vi "WriteSystemData.vi"(8 "error in (no error)":errorcluster, 10 "SystemData":T1 {"SourceSelect" items=["儀器1"]}, 11 "DataNotifierIn":refnum<notifier>) -> (0 "error out":errorcluster, 3 "DataNotifierOut":refnum<notifier>)   [LabVIEW 2013, in "SystemData.lvclass"]
uses:
  SystemData.lvclass
  SystemDataTypeDefine.ctl
  Generator.lvclass/Generator.lvclass
  SystemData.lvclass/SystemData.ctl
panel:
  # "以notifier包裝systemData物件的參考\n如此不論在何處只要輸入正確notifier 參考\n就可以正確提出systemData物件保存的資料"
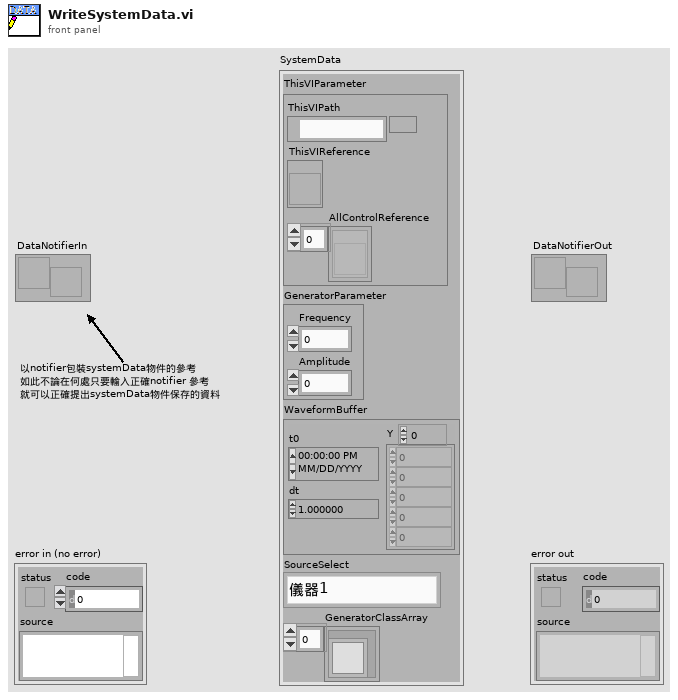
[diagram p1: front panel]
types:
  T1 = typedef "SystemData.lvclass/SystemDataTypeDefine.ctl" = cluster{"ThisVIParameter":cluster{"ThisVIPath":path, "ThisVIReference":refnum<vi>, "AllControlReference":refnum<vi>[]}, "GeneratorParameter":cluster{"Frequency":dbl, "Amplitude":dbl}, "WaveformBuffer":waveform(dbl), "SourceSelect":u16, "GeneratorClassArray":refnum<class "Generator.lvclass">[]}
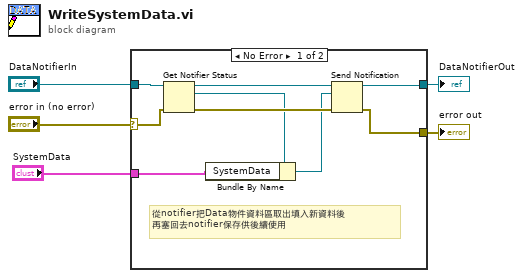
[diagram p0: block diagram]
diagram:
  n1 = case shown="No Error" "error in (no error)" {
    selector: "error in (no error)" -> [w10 w15]
    tunnel: [w9 w15] -> w4
    tunnel: [w11 w16] -> w2
    tunnel: "DataNotifierIn" -> [w14 w16]
    tunnel: "SystemData" -> [w7 _]
    frame No Error {
      # "從notifier把Data物件資料區取出填入新資料後\n再塞回去notifier保存供後續使用"
      n2 = Get Notifier Status(notifier=w14, error in (no error)=w10) -> (notifier out=w13:refnum<notifier>, current notification=w8:refnum<class "SystemData.lvclass">, error out=w12:errorcluster)  [unwired: 2 out]
      n3 = Bundle By Name(cluster=w8, "SystemData"=w7) -> (w6:refnum<class "SystemData.lvclass">)
      n4 = Send Notification(notification=w6, notifier=w13, error in (no error)=w12) -> (notifier out=w11:refnum<notifier>, error out=w9:errorcluster)
    }
    frame Error {
    }
  }
  "error out" <- w4
  "DataNotifierOut" <- w2
